vi "Event Loop.vi"(11 "Event Loop in":refnum<class "Event Loop.lvclass">) -> (3 "Event Loop out":refnum<class "Event Loop.lvclass">)   [LabVIEW 2021, in "Event Loop.lvlib" / "Event Loop.lvclass"]
uses:
  Event Loop.lvclass
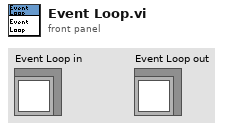
[diagram p1: front panel]
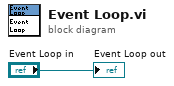
[diagram p0: block diagram]
diagram:
  "Event Loop out" <- "Event Loop in"
